vi "Open Arguments UI.vi"(5 "Title":string="Error Arguments Window", 7 "Path":path=path "Error Arguments Window.vi", 8 "error in":errorcluster, 10 "Calling VI Ref":refnum<vi>, 11 "App Instance":refnum<vi>) -> (0 "error out":errorcluster, 3 "Error Arguments Window Ref":refnum<vi>)   [LabVIEW 2020, in "ConstantErrorsMaker.lvlib"]
uses:
  ConstantErrorsMaker.lvlib
  <vilib>/Utility/miscctls.llb/LVRectTypeDef.ctl
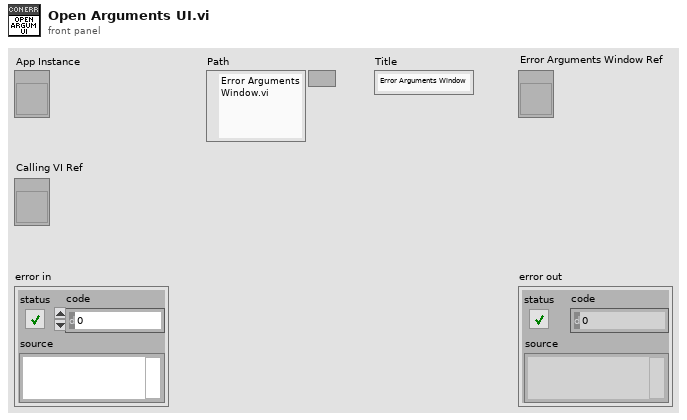
[diagram p1: front panel]
types:
  T1 = typedef "LVRectTypeDef.ctl" = cluster{"Left":i16, "Top":i16, "Right":i16, "Bottom":i16}
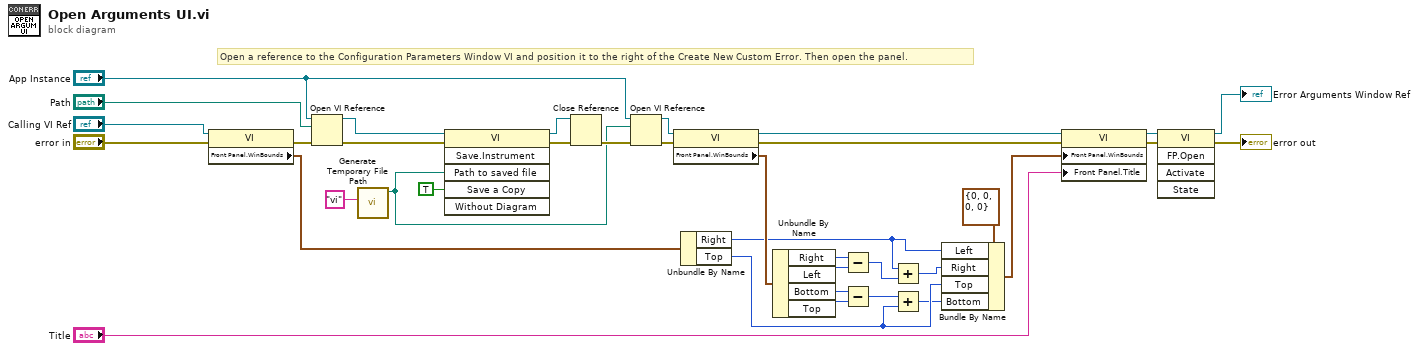
[diagram p0: block diagram]
diagram:
  # "Open a reference to the Configuration Parameters Window VI and position it to the right of the Create New Custom Error. Then open the panel."
  n1 = property class="VI"(reference="Calling VI Ref", error in="error in") -> (error out=w28:errorcluster, "Front Panel.WinBounds"=w1:T1)  [unwired: 1 out]
  n2 = Open VI Reference(application reference (local)="App Instance", vi path="Path", error in (no error)=w28) -> (vi reference=w9:refnum<vi>, error out=w34:errorcluster)  [unwired: 3 in]
  n3 = call <vilib>:"Generate Temporary File Path.vi"("Temporary File Extension (tmp)"="vi") -> ("Unique Temporary File Path"=w4:path)  [unwired: 9 in, 1 out]
  n4 = invoke class="VI" method="Save.Instrument"(reference=w9, error in=w34, "Path to saved file"=w4, "Save a Copy"=TRUE) -> (reference out=w6:refnum<vi>, error out=w33:errorcluster)  [unwired: 2 in, 4 out]
  n5 = Close Reference(reference=w6, error in (no error)=w33) -> (error out=w32:errorcluster)
  n6 = Open VI Reference(application reference (local)="App Instance", vi path=w4, error in (no error)=w32) -> (vi reference=w5:refnum<vi>, error out=w31:errorcluster)  [unwired: 3 in]
  n7 = property class="VI"(reference=w5, error in=w31) -> (reference out=w24:refnum<vi>, error out=w35:errorcluster, "Front Panel.WinBounds"=w21:T1)
  n8 = Unbundle By Name(w1) -> ("Right"=w12:i16, "Top"=w15:i16)
  n9 = Unbundle By Name(w21) -> ("Right"=w20:i16, "Left"=w19:i16, "Bottom"=w18:i16, "Top"=w17:i16)
  n10 = Subtract(x=w20, y=w19) -> (x-y=w11:i16)
  n11 = Subtract(x=w18, y=w17) -> (x-y=w16:i16)
  n12 = Add(x=w12, y=w11) -> (x+y=w13:i16)
  n13 = Add(x=w16, y=w15) -> (x+y=w14:i16)
  n14 = Bundle By Name(cluster=T1 {"Left"=0, "Top"=0, "Right"=0, "Bottom"=0} ("Front Panel Window:Window Bounds"), "Left"=w12, "Right"=w13, "Top"=w15, "Bottom"=w14) -> (w22:T1)
  n15 = property class="VI"(reference=w24, error in=w35, "Front Panel.WinBounds"=w22, "Front Panel.Title"="Title") -> (reference out=w26:refnum<vi>, error out=w36:errorcluster)
  n16 = invoke class="VI" method="FP.Open"(reference=w26, error in=w36) -> (reference out=→"Error Arguments Window Ref":refnum<vi>, error out=→"error out":errorcluster)  [unwired: 3 in, 3 out]
